vi "Seebeck.vi"() -> ()   [LabVIEW 2024]
uses:
  <vilib>/express/express shared/transition.llb/Dynamic To Waveform Array.vi
  <vilib>/express/express signal manip/GetorSetDDTAttributes/Set DDT Attributes/SetT0.vi
  <vilib>/express/express shared/transition.llb/Waveform Array To Dynamic.vi
  <vilib>/express/express signal manip/GetorSetDDTAttributes/Set DDT Attributes/Set DDT Properties.xnode
  <instrlib>/Arduino UNO/Arduino UNO.lvlib
  <instrlib>/BK Precision 5491B/BK Precision 5491B.lvlib
panel:
  out "Temperature L":dbl
  out "Temperature 2":string
  in  "Secondary Function (1: AC Volts)":u16(ring)=1 items=["DC Volts", "AC Volts", "DC Current", "AC Current", "Frequency", "dB", "dBm"]
  in  "Auto Range (T:Enable)":bool=TRUE
  in  "Manual Range (1000)":dbl=1000.0 format="%#.3f"
  in  "Primary Function (0: DC Volts)":u16(ring) items=["DC Volts", "AC Volts", "AC+DC Volts", "DC Current", "AC Current", "AC+DC Current", "2-Wire Resistance", "Frequency", "Period", "Diode", "Continuity"]
  in  "Serial Configuration":T1={"Baud Rate"=9600, "Parity"=0, "Data Bits"=8, "Stop Bits"=10, "Flow Control"=0} {"Flow Control" items=["None", "XON/XOFF", "RTS/CTS", "XON/XOFF & RTS/CTS", "DTR/DSR", "XON/XOFF & DTR/DSR"]; "Stop Bits" items=["1.0"=10, "1.5"=15, "2.0"=20]; "Data Bits" items=["8"=8]; "Parity" items=["None", "Odd", "Even", "Mark", "Space"]; "Baud Rate" items=["4800"=4800, "9600"=9600, "19200"=19200, "38400"=38400]}
  in  "VISA resource name 3":refnum<visa-resource-name>
  out "Secondary Measurement":dbl
  out "Primary Measurement":dbl
  in  "stop":bool
  out "Temperature H":dbl
  in  "VISA resource name":refnum<visa-resource-name>
  out "Temperature":string
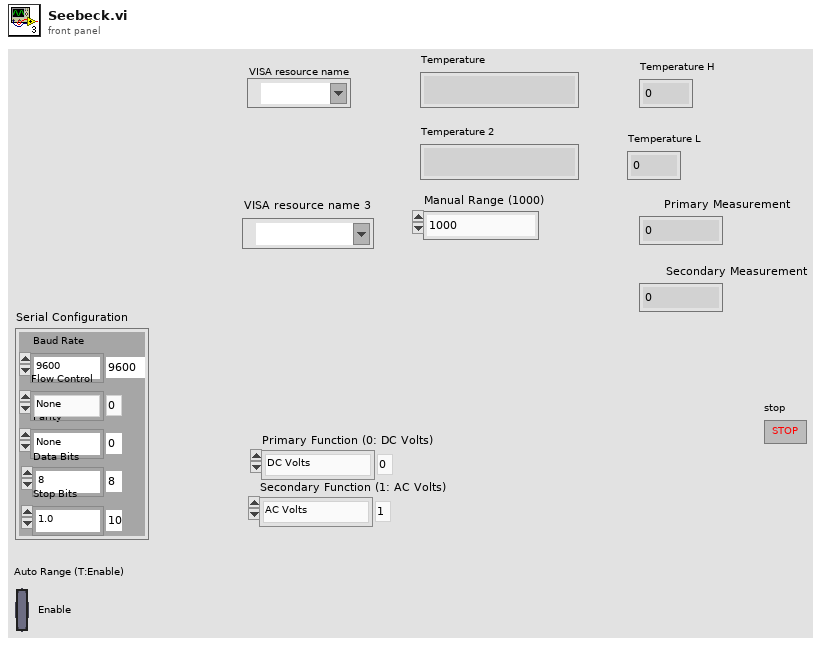
[diagram p1: front panel]
types:
  T1 = cluster{"Baud Rate":u32, "Parity":u16, "Data Bits":u16, "Stop Bits":u16, "Flow Control":u16}
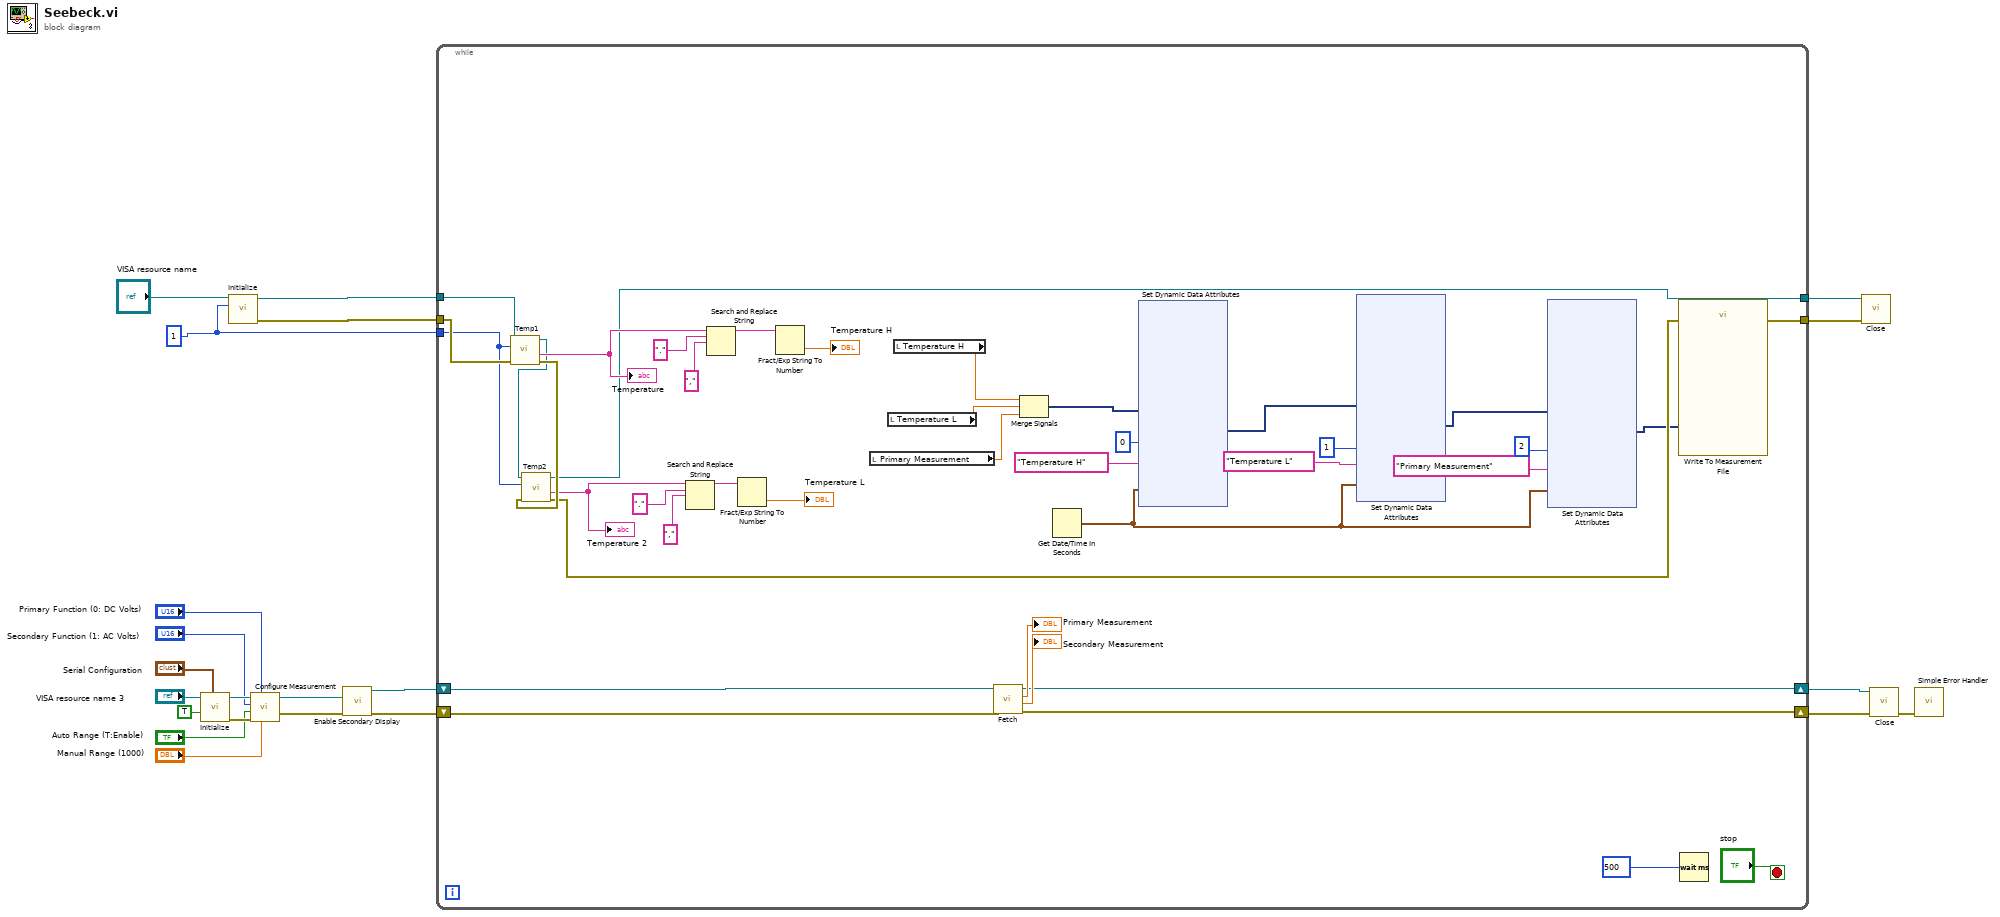
[diagram p0: block diagram]
diagram:
  w17 = 1
  n1 = call <instrlib>:"Initialize.vi"("Serial Configuration"="Serial Configuration", "Reset (True)"=TRUE, "VISA resource name"="VISA resource name 3") -> ("error out"=w14:errorcluster, "VISA resource name out"=w15:refnum<visa-resource-name>)  [unwired: 7 in]
  n2 = call <instrlib>:"Initialize.vi"("Address"=w17, "VISA resource name"="VISA resource name") -> ("error IO"=w19:errorcluster, "VISA resource name out"=w18:refnum<visa-resource-name>)  [unwired: 7 in, 1 out]
  n3 = call <instrlib>:"Configure Measurement.vi"("Manual Range (1000)"="Manual Range (1000)", "Primary Function (0: DC Volts)"="Primary Function (0: DC Volts)", "error in (no error)"=w14, "Auto Range (T:Enable)"="Auto Range (T:Enable)", "Secondary Function (1: AC Volts)"="Secondary Function (1: AC Volts)", "VISA resource name"=w15) -> ("error out"=w6:errorcluster, "VISA resource name out"=w7:refnum<visa-resource-name>)  [unwired: 4 in]
  n4 = call <instrlib>:"Enable Secondary Display.vi"("error in (no error)"=w6, "VISA resource name"=w7) -> ("error out"=w4:errorcluster, "VISA resource name out"=w5:refnum<visa-resource-name>)  [unwired: 8 in]
  n5 = while {
    tunnel: [w30] -> w22
    tunnel: [w29] -> w21
    tunnel: w19 -> [w40]
    tunnel: w18 -> [w41]
    tunnel: w17 -> [w36]
    shift-right: [w43] -> w2
    shift-left: w5 -> [w45]
    shift-right: [w42] -> w1
    shift-left: w4 -> [w44]
    stop <- "stop" stop-if-true
    n6 = call <instrlib>:"Temp1.vi"("error in (no error)"=w40, "Address"=w36, "VISA resource name"=w41) -> ("error IO"=w38:errorcluster, "Pressure"=w39:string, "VISA resource name out"=w37:refnum<visa-resource-name>)  [unwired: 6 in]
    "Temperature" <- w39
    n7 = call <instrlib>:"Temp2.vi"("error in (no error)"=w38, "Address"=w36, "VISA resource name"=w37) -> ("error IO"=w29:errorcluster, "Pressure"=w32:string, "VISA resource name out"=w30:refnum<visa-resource-name>)  [unwired: 6 in]
    "Temperature 2" <- w32
    n8 = Search and Replace String(input string=w32, search string=".", replace string=",") -> (result string=w33:string)  [unwired: 5 in, 3 out]
    n9 = Search and Replace String(input string=w39, search string=".", replace string=",") -> (result string=w59:string)  [unwired: 5 in, 3 out]
    n10 = Fract/Exp String To Number(string=w33) -> (number=→"Temperature L":dbl)  [unwired: 3 in, 1 out]
    n11 = Fract/Exp String To Number(string=w59) -> (number=→"Temperature H":dbl)  [unwired: 3 in, 1 out]
    n12 = local read "Primary Measurement"() -> (w28:dbl)
    n13 = local read "Temperature L"() -> (w56:dbl)
    n14 = local read "Temperature H"() -> (w57:dbl)
    n15 = call <instrlib>:"Fetch.vi"("error in (no error)"=w44, "VISA resource name"=w45) -> ("error out"=w42:errorcluster, "Secondary Measurement"=→"Secondary Measurement":dbl, "Primary Measurement"=→"Primary Measurement":dbl, "VISA resource name out"=w43:refnum<visa-resource-name>)  [unwired: 6 in]
    n16 = Merge Signals(w57, w56, w28) -> (w55:dynamicdata)
    n17 = Get Date/Time In Seconds() -> (seconds since 1Jan1904=w27:timestamp)
    n18 = xnode "Set Dynamic Data Attributes"("Signals In"=w55, "Signal Index"=0, "Signal Name"="Temperature H", "Timestamp"=w27) -> ("Signals Out"=w52:dynamicdata)  [unwired: 1 in, 1 out]
    n19 = xnode "Set Dynamic Data Attributes"("Signals In"=w52, "Signal Index"=1, "Signal Name"="Temperature L", "Timestamp"=w27) -> ("Signals Out"=w24:dynamicdata)  [unwired: 1 in, 1 out]
    n20 = xnode "Set Dynamic Data Attributes"("Signals In"=w24, "Signal Index"=2, "Signal Name"="Primary Measurement", "Timestamp"=w27) -> ("Signals Out"=w23:dynamicdata)  [unwired: 1 in, 1 out]
    n21 = call "Write To Measurement File"("Signals"=w23) -> ()  [unwired: 16 in, 3 out]
    n22 = Wait (ms)(milliseconds to wait=u32 500) -> ()  [unwired: 1 out]
  }
  n23 = call <instrlib>:"Close.vi"("error in (no error)"=w21, "VISA resource name"=w22) -> ()  [unwired: 9 in, 1 out]
  n24 = call <instrlib>:"Close.vi"("error in (no error)"=w1, "VISA resource name"=w2) -> ("error out"=w3:errorcluster)  [unwired: 9 in]
  n25 = call <vilib>:"Simple Error Handler.vi"("error in (no error)"=w3) -> ()  [unwired: 4 in, 5 out]
